vi "Send Go_to_Idle.vi"(7 "Message Priority (Normal)":T1=enum."Normal", 8 "error in (no error)":errorcluster, 10 "Nested in":refnum<class "ATM_UI_Controller.lvclass">, 11 "Message Enqueuer":refnum<class "Message Enqueuer.lvclass">) -> (0 "error out":errorcluster, 3 "Message Enqueuer out":refnum<class "Message Enqueuer.lvclass">)   [LabVIEW 2025, in "User_Console.lvlib" / "Go_to_Idle Msg.lvclass"]
doc: "This VI sends the message to an actor."
uses:
  Go_to_Idle Msg.lvclass
  <vilib>/ActorFramework/Message Enqueuer/Message Enqueuer.lvclass
  <vilib>/ActorFramework/Message Enqueuer/Message Priority.ctl
  ATM_UI_Controller/ATM_UI_Controller.lvclass
  C:/Program Files (x86)/National Instruments/LabVIEW 2025/vi.lib/ActorFramework/Message/Message.lvclass
  Go_to_Idle Msg.lvclass/Go_to_Idle Msg.ctl
  <vilib>/ActorFramework/Message Enqueuer/Message Enqueuer.lvclass/Message Enqueuer.ctl
  <vilib>/ActorFramework/Message Priority Queue/Priority Enqueue.vi
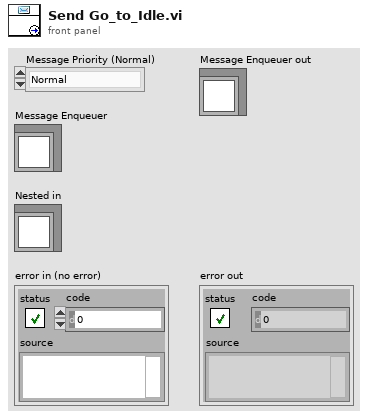
[diagram p1: front panel]
types:
  T1 = typedef "Actor Framework.lvlib/Message Enqueuer.lvclass/Message Priority.ctl" = enum16{"Low", "Normal", "High"}
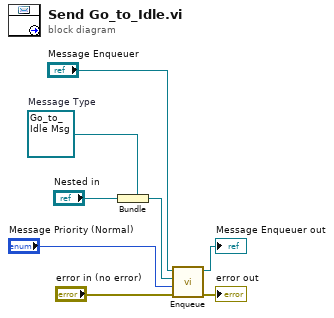
[diagram p0: block diagram]
diagram:
  w2 = refnum<class "Go_to_Idle Msg.lvclass"> refnum  # Message Type
  n1 = Bundle(cluster=w2, "Nested in") -> (w3:refnum<class "Go_to_Idle Msg.lvclass">)
  n2 = call <vilib>:"Enqueue.vi"("error in (no error)"="error in (no error)", "Message Priority (Normal)"="Message Priority (Normal)", "Message"=w3, "Message Enqueuer in"="Message Enqueuer") -> ("error out"=→"error out":errorcluster, "Message Enqueuer out"=→"Message Enqueuer out":refnum<class "Message Enqueuer.lvclass">)  [unwired: 6 in]
